vi "输入数据解析.vi"(0 "单个参数补充":dbl, 1 "从板号":dbl=1.0, 2 "主板二维码":string="BNET01", 3 "从板二维码":string="BNET01", 5 "主板引用":refnum<vi>, 7 "从板引用":refnum<vi>, 9 "主板选项":string="三级故障阀值", 11 "枚举":enum16{"主板", "从板"}(ring), 12 "快换":bool caption="快换写入") -> (4 "输出数组":dbl[][](array[numeric]), 6 "数组长度":dbl[](array[numeric]), 8 "循环次数":i32, 10 "命令":u32, 14 "名称":string[](array[string]), 15 "命令序号":u32[](array[numeric]))   [LabVIEW 2013] (continued)
              tunnel: [w18498 w18509 w18520 w18531 w18541 w18551 w18562] -> w18492
              frame 0, Default {
                # "电压过高"
                n7256 = disable-structure shown="启用" {
                  disable-tunnel: [w18504 w18507] -> w18500
                  disable-tunnel: [w18503 w18507] -> w18499
                  disable-tunnel: w18497 -> [w18502 _]
                  frame Disabled {
                    n7257 = Unbundle By Name(w18502) -> ("电压过高"=w18501:dbl)
                    n7258 = call "输入分辨率计算-EV05.vi"("1字节?"=FALSE, "数值"=w18501, "分辨率"=0.1) -> ("低字节"=w18503:dbl, "高字节1"=w18504:dbl)  [unwired: 2 in, 5 out]
                  }
                  frame Enabled {
                    w18507 = 255 ("高字节1")
                  }
                }
                n7259 = Build Array(w18500, w18499) -> (w18498:i32[])
              }
              frame 1 {
                # "电压过低"
                n7260 = disable-structure shown="启用" {
                  disable-tunnel: [w18515 w18518] -> w18511
                  disable-tunnel: [w18514 w18518] -> w18510
                  disable-tunnel: w18508 -> [w18513 _]
                  frame Disabled {
                    n7261 = Unbundle By Name(w18513) -> ("电压过低"=w18512:dbl)
                    n7262 = call "输入分辨率计算-EV05.vi"("1字节?"=FALSE, "数值"=w18512, "分辨率"=0.1) -> ("低字节"=w18514:dbl, "高字节1"=w18515:dbl)  [unwired: 2 in, 5 out]
                  }
                  frame Enabled {
                    w18518 = 255 ("高字节1")
                  }
                }
                n7263 = Build Array(w18511, w18510) -> (w18509:i32[])
              }
              frame 2 {
                # "电压不均衡"
                n7264 = disable-structure shown="启用" {
                  disable-tunnel: [w18526 w18529] -> w18522
                  disable-tunnel: [w18525 w18529] -> w18521
                  disable-tunnel: w18519 -> [w18524 _]
                  frame Disabled {
                    n7265 = Unbundle By Name(w18524) -> ("电压不均衡(V)"=w18523:dbl)
                    n7266 = call "输入分辨率计算-EV05.vi"("1字节?"=FALSE, "数值"=w18523, "分辨率"=0.1) -> ("低字节"=w18525:dbl, "高字节1"=w18526:dbl)  [unwired: 2 in, 5 out]
                  }
                  frame Enabled {
                    w18529 = 255 ("高字节1")
                  }
                }
                n7267 = Build Array(w18522, w18521) -> (w18520:i32[])
              }
              frame 3 {
                # "温度过高"
                n7268 = disable-structure shown="启用" {
                  disable-tunnel: [w18536 255 ("高字节1")] -> w18532
                  disable-tunnel: w18530 -> [w18534 _]
                  frame Disabled {
                    n7269 = Unbundle By Name(w18534) -> ("温度过高"=w18533:dbl)
                    n7270 = call "输入分辨率计算-EV05.vi"("1字节?"=TRUE, "数值"=w18533, "偏移量"=-40.0, "分辨率"=1.0) -> ("高字节1"=w18536:dbl)  [unwired: 1 in, 6 out]
                  }
                  frame Enabled {
                  }
                }
                n7271 = Build Array(w18532) -> (w18531:i32[])
              }
              frame 4 {
                # "温度过低"
                n7272 = disable-structure shown="启用" {
                  disable-tunnel: [w18546 255 ("高字节1")] -> w18542
                  disable-tunnel: w18540 -> [w18544 _]
                  frame Disabled {
                    n7273 = Unbundle By Name(w18544) -> ("温度过低"=w18543:dbl)
                    n7274 = call "输入分辨率计算-EV05.vi"("1字节?"=TRUE, "数值"=w18543, "偏移量"=-40.0, "分辨率"=1.0) -> ("高字节1"=w18546:dbl)  [unwired: 1 in, 6 out]
                  }
                  frame Enabled {
                  }
                }
                n7275 = Build Array(w18542) -> (w18541:i32[])
              }
              frame 5 {
                # "温度不均衡"
                n7276 = disable-structure shown="启用" {
                  disable-tunnel: [w18555 255 ("高字节1")] -> w18552
                  disable-tunnel: w18550 -> [w18554 _]
                  frame Disabled {
                    n7277 = Unbundle By Name(w18554) -> ("温度不均衡"=w18553:dbl)
                    n7278 = call "输入分辨率计算-EV05.vi"("1字节?"=TRUE, "数值"=w18553, "分辨率"=1.0) -> ("高字节1"=w18555:dbl)  [unwired: 2 in, 6 out]
                  }
                  frame Enabled {
                  }
                }
                n7279 = Build Array(w18552) -> (w18551:i32[])
              }
              frame 6 {
                # "SOC过低"
                n7280 = disable-structure shown="启用" {
                  disable-tunnel: w18561 -> [w18566 _]
                  disable-tunnel: [w18563 w18569] -> w18560
                  disable-tunnel: [w18564 w18569] -> w18559
                  frame Enabled {
                    n7281 = Unbundle By Name(w18566) -> ("SOC过低"=w18565:dbl)
                    n7282 = call "输入分辨率计算-EV05.vi"("1字节?"=FALSE, "数值"=w18565, "分辨率"=0.1) -> ("低字节"=w18563:dbl, "高字节1"=w18564:dbl)  [unwired: 2 in, 5 out]
                  }
                  frame Disabled {
                    w18569 = 255 ("高字节1")
                  }
                }
                n7283 = Build Array(w18559, w18560) -> (w18562:dbl[])
              }
            }
            n7284 = Insert Into Array(array=w18493, new element=w18492) -> (w18494:dbl[])  [unwired: 1 in]
          }
          n7285 = Build Array(w18487) -> (w18486:dbl[][])
        }
        frame "SOC过低(2)" {
          n7286 = Unbundle By Name(w18574) -> ("二级故障(从板)"=w18575:refnum<vi>)
          n7287 = property class="Clust (严格)"(reference=w18575) -> ("Value"=w18573:T8)  [unwired: 1 in, 2 out]
          n7288 = for {
            N: 7 -> [_]
            tunnel: w18573 -> [w18585]
            shift-right: [w18584] -> w18577
            shift-left: dbl[] [] -> [w18583]
            i -> [w18586]
            n7289 = case shown="6" w18586 {
              tunnel: w18585 -> [w18587 w18598 w18609 w18620 w18630 w18640 w18651]
              tunnel: [w18588 w18599 w18610 w18621 w18631 w18641 w18652] -> w18582
              frame 0, Default {
                # "电压过高"
                n7290 = disable-structure shown="启用" {
                  disable-tunnel: [w18594 w18597] -> w18590
                  disable-tunnel: [w18593 w18597] -> w18589
                  disable-tunnel: w18587 -> [w18592 _]
                  frame Disabled {
                    n7291 = Unbundle By Name(w18592) -> ("电压过高"=w18591:dbl)
                    n7292 = call "输入分辨率计算-EV05.vi"("1字节?"=FALSE, "数值"=w18591, "分辨率"=0.1) -> ("低字节"=w18593:dbl, "高字节1"=w18594:dbl)  [unwired: 2 in, 5 out]
                  }
                  frame Enabled {
                    w18597 = 255 ("高字节1")
                  }
                }
                n7293 = Build Array(w18590, w18589) -> (w18588:i32[])
              }
              frame 1 {
                # "电压过低"
                n7294 = disable-structure shown="启用" {
                  disable-tunnel: [w18605 w18608] -> w18601
                  disable-tunnel: [w18604 w18608] -> w18600
                  disable-tunnel: w18598 -> [w18603 _]
                  frame Disabled {
                    n7295 = Unbundle By Name(w18603) -> ("电压过低"=w18602:dbl)
                    n7296 = call "输入分辨率计算-EV05.vi"("1字节?"=FALSE, "数值"=w18602, "分辨率"=0.1) -> ("低字节"=w18604:dbl, "高字节1"=w18605:dbl)  [unwired: 2 in, 5 out]
                  }
                  frame Enabled {
                    w18608 = 255 ("高字节1")
                  }
                }
                n7297 = Build Array(w18601, w18600) -> (w18599:i32[])
              }
              frame 2 {
                # "电压不均衡"
                n7298 = disable-structure shown="启用" {
                  disable-tunnel: [w18616 w18619] -> w18612
                  disable-tunnel: [w18615 w18619] -> w18611
                  disable-tunnel: w18609 -> [w18614 _]
                  frame Disabled {
                    n7299 = Unbundle By Name(w18614) -> ("电压不均衡(V)"=w18613:dbl)
                    n7300 = call "输入分辨率计算-EV05.vi"("1字节?"=FALSE, "数值"=w18613, "分辨率"=0.1) -> ("低字节"=w18615:dbl, "高字节1"=w18616:dbl)  [unwired: 2 in, 5 out]
                  }
                  frame Enabled {
                    w18619 = 255 ("高字节1")
                  }
                }
                n7301 = Build Array(w18612, w18611) -> (w18610:i32[])
              }
              frame 3 {
                # "温度过高"
                n7302 = disable-structure shown="启用" {
                  disable-tunnel: [w18626 255 ("高字节1")] -> w18622
                  disable-tunnel: w18620 -> [w18624 _]
                  frame Disabled {
                    n7303 = Unbundle By Name(w18624) -> ("温度过高"=w18623:dbl)
                    n7304 = call "输入分辨率计算-EV05.vi"("1字节?"=TRUE, "数值"=w18623, "偏移量"=-40.0, "分辨率"=1.0) -> ("高字节1"=w18626:dbl)  [unwired: 1 in, 6 out]
                  }
                  frame Enabled {
                  }
                }
                n7305 = Build Array(w18622) -> (w18621:i32[])
              }
              frame 4 {
                # "温度过低"
                n7306 = disable-structure shown="启用" {
                  disable-tunnel: [w18636 255 ("高字节1")] -> w18632
                  disable-tunnel: w18630 -> [w18634 _]
                  frame Disabled {
                    n7307 = Unbundle By Name(w18634) -> ("温度过低"=w18633:dbl)
                    n7308 = call "输入分辨率计算-EV05.vi"("1字节?"=TRUE, "数值"=w18633, "偏移量"=-40.0, "分辨率"=1.0) -> ("高字节1"=w18636:dbl)  [unwired: 1 in, 6 out]
                  }
                  frame Enabled {
                  }
                }
                n7309 = Build Array(w18632) -> (w18631:i32[])
              }
              frame 5 {
                # "温度不均衡"
                n7310 = disable-structure shown="启用" {
                  disable-tunnel: [w18645 255 ("高字节1")] -> w18642
                  disable-tunnel: w18640 -> [w18644 _]
                  frame Disabled {
                    n7311 = Unbundle By Name(w18644) -> ("温度不均衡"=w18643:dbl)
                    n7312 = call "输入分辨率计算-EV05.vi"("1字节?"=TRUE, "数值"=w18643, "分辨率"=1.0) -> ("高字节1"=w18645:dbl)  [unwired: 2 in, 6 out]
                  }
                  frame Enabled {
                  }
                }
                n7313 = Build Array(w18642) -> (w18641:i32[])
              }
              frame 6 {
                # "SOC过低"
                n7314 = disable-structure shown="启用" {
                  disable-tunnel: w18651 -> [w18656 _]
                  disable-tunnel: [w18653 w18659] -> w18650
                  disable-tunnel: [w18654 w18659] -> w18649
                  frame Enabled {
                    n7315 = Unbundle By Name(w18656) -> ("SOC过低"=w18655:dbl)
                    n7316 = call "输入分辨率计算-EV05.vi"("1字节?"=FALSE, "数值"=w18655, "分辨率"=0.1) -> ("低字节"=w18653:dbl, "高字节1"=w18654:dbl)  [unwired: 2 in, 5 out]
                  }
                  frame Disabled {
                    w18659 = 255 ("高字节1")
                  }
                }
                n7317 = Build Array(w18649, w18650) -> (w18652:dbl[])
              }
            }
            n7318 = Insert Into Array(array=w18583, new element=w18582) -> (w18584:dbl[])  [unwired: 1 in]
          }
          n7319 = Build Array(w18577) -> (w18576:dbl[][])
        }
        frame "SOC过低(3)" {
          n7320 = Unbundle By Name(w18664) -> ("三级故障(从板)"=w18665:refnum<vi>)
          n7321 = property class="Clust (严格)"(reference=w18665) -> ("Value"=w18663:T8)  [unwired: 1 in, 2 out]
          n7322 = for {
            N: 7 -> [_]
            tunnel: w18663 -> [w18675]
            shift-right: [w18674] -> w18667
            shift-left: dbl[] [] -> [w18673]
            i -> [w18676]
            n7323 = case shown="6" w18676 {
              tunnel: w18675 -> [w18677 w18688 w18699 w18710 w18720 w18730 w18741]
              tunnel: [w18678 w18689 w18700 w18711 w18721 w18731 w18742] -> w18672
              frame 0, Default {
                # "电压过高"
                n7324 = disable-structure shown="启用" {
                  disable-tunnel: [w18684 w18687] -> w18680
                  disable-tunnel: [w18683 w18687] -> w18679
                  disable-tunnel: w18677 -> [w18682 _]
                  frame Disabled {
                    n7325 = Unbundle By Name(w18682) -> ("电压过高"=w18681:dbl)
                    n7326 = call "输入分辨率计算-EV05.vi"("1字节?"=FALSE, "数值"=w18681, "分辨率"=0.1) -> ("低字节"=w18683:dbl, "高字节1"=w18684:dbl)  [unwired: 2 in, 5 out]
                  }
                  frame Enabled {
                    w18687 = 255 ("高字节1")
                  }
                }
                n7327 = Build Array(w18680, w18679) -> (w18678:i32[])
              }
              frame 1 {
                # "电压过低"
                n7328 = disable-structure shown="启用" {
                  disable-tunnel: [w18695 w18698] -> w18691
                  disable-tunnel: [w18694 w18698] -> w18690
                  disable-tunnel: w18688 -> [w18693 _]
                  frame Disabled {
                    n7329 = Unbundle By Name(w18693) -> ("电压过低"=w18692:dbl)
                    n7330 = call "输入分辨率计算-EV05.vi"("1字节?"=FALSE, "数值"=w18692, "分辨率"=0.1) -> ("低字节"=w18694:dbl, "高字节1"=w18695:dbl)  [unwired: 2 in, 5 out]
                  }
                  frame Enabled {
                    w18698 = 255 ("高字节1")
                  }
                }
                n7331 = Build Array(w18691, w18690) -> (w18689:i32[])
              }
              frame 2 {
                # "电压不均衡"
                n7332 = disable-structure shown="启用" {
                  disable-tunnel: [w18706 w18709] -> w18702
                  disable-tunnel: [w18705 w18709] -> w18701
                  disable-tunnel: w18699 -> [w18704 _]
                  frame Disabled {
                    n7333 = Unbundle By Name(w18704) -> ("电压不均衡(V)"=w18703:dbl)
                    n7334 = call "输入分辨率计算-EV05.vi"("1字节?"=FALSE, "数值"=w18703, "分辨率"=0.1) -> ("低字节"=w18705:dbl, "高字节1"=w18706:dbl)  [unwired: 2 in, 5 out]
                  }
                  frame Enabled {
                    w18709 = 255 ("高字节1")
                  }
                }
                n7335 = Build Array(w18702, w18701) -> (w18700:i32[])
              }
              frame 3 {
                # "温度过高"
                n7336 = disable-structure shown="启用" {
                  disable-tunnel: [w18716 255 ("高字节1")] -> w18712
                  disable-tunnel: w18710 -> [w18714 _]
                  frame Disabled {
                    n7337 = Unbundle By Name(w18714) -> ("温度过高"=w18713:dbl)
                    n7338 = call "输入分辨率计算-EV05.vi"("1字节?"=TRUE, "数值"=w18713, "偏移量"=-40.0, "分辨率"=1.0) -> ("高字节1"=w18716:dbl)  [unwired: 1 in, 6 out]
                  }
                  frame Enabled {
                  }
                }
                n7339 = Build Array(w18712) -> (w18711:i32[])
              }
              frame 4 {
                # "温度过低"
                n7340 = disable-structure shown="启用" {
                  disable-tunnel: [w18726 255 ("高字节1")] -> w18722
                  disable-tunnel: w18720 -> [w18724 _]
                  frame Disabled {
                    n7341 = Unbundle By Name(w18724) -> ("温度过低"=w18723:dbl)
                    n7342 = call "输入分辨率计算-EV05.vi"("1字节?"=TRUE, "数值"=w18723, "偏移量"=-40.0, "分辨率"=1.0) -> ("高字节1"=w18726:dbl)  [unwired: 1 in, 6 out]
                  }
                  frame Enabled {
                  }
                }
                n7343 = Build Array(w18722) -> (w18721:i32[])
              }
              frame 5 {
                # "温度不均衡"
                n7344 = disable-structure shown="启用" {
                  disable-tunnel: [w18735 255 ("高字节1")] -> w18732
                  disable-tunnel: w18730 -> [w18734 _]
                  frame Disabled {
                    n7345 = Unbundle By Name(w18734) -> ("温度不均衡"=w18733:dbl)
                    n7346 = call "输入分辨率计算-EV05.vi"("1字节?"=TRUE, "数值"=w18733, "分辨率"=1.0) -> ("高字节1"=w18735:dbl)  [unwired: 2 in, 6 out]
                  }
                  frame Enabled {
                  }
                }
                n7347 = Build Array(w18732) -> (w18731:i32[])
              }
              frame 6 {
                # "SOC过低"
                n7348 = disable-structure shown="启用" {
                  disable-tunnel: w18741 -> [w18746 _]
                  disable-tunnel: [w18743 w18749] -> w18740
                  disable-tunnel: [w18744 w18749] -> w18739
                  frame Enabled {
                    n7349 = Unbundle By Name(w18746) -> ("SOC过低"=w18745:dbl)
                    n7350 = call "输入分辨率计算-EV05.vi"("1字节?"=FALSE, "数值"=w18745, "分辨率"=0.1) -> ("低字节"=w18743:dbl, "高字节1"=w18744:dbl)  [unwired: 2 in, 5 out]
                  }
                  frame Disabled {
                    w18749 = 255 ("高字节1")
                  }
                }
                n7351 = Build Array(w18739, w18740) -> (w18742:dbl[])
              }
            }
            n7352 = Insert Into Array(array=w18673, new element=w18672) -> (w18674:dbl[])  [unwired: 1 in]
          }
          n7353 = Build Array(w18667) -> (w18666:dbl[][])
        }
        frame "二级故障阀值" {
          n7354 = Unbundle By Name(w18754) -> ("二级故障(从板)"=w18755:refnum<vi>)
          n7355 = property class="Clust (严格)"(reference=w18755) -> ("Value"=w18753:T8)  [unwired: 1 in, 2 out]
          n7356 = for {
            N: 7 -> [_]
            tunnel: w18753 -> [w18765]
            shift-right: [w18764] -> w18757
            shift-left: dbl[] [] -> [w18763]
            i -> [w18766]
            n7357 = case shown="5" w18766 {
              tunnel: w18765 -> [w18768 w18775 w18782 w18789 w18796 w18803 w18811]
              tunnel: [w18769 w18776 w18783 w18791 w18798 w18804 w18812] -> w18762
              frame 0, Default {
                # "电压过高"
                n7358 = Unbundle By Name(w18768) -> ("电压过高"=w18767:dbl)
                n7359 = call "输入分辨率计算-EV05.vi"("1字节?"=FALSE, "数值"=w18767, "分辨率"=0.001) -> ("低字节"=w18770:dbl, "高字节1"=w18771:dbl)  [unwired: 2 in, 5 out]
                n7360 = Build Array(w18771, w18770) -> (w18769:dbl[])
              }
              frame 1 {
                # "电压过低"
                n7361 = Unbundle By Name(w18775) -> ("电压过低"=w18774:dbl)
                n7362 = call "输入分辨率计算-EV05.vi"("1字节?"=FALSE, "数值"=w18774, "分辨率"=0.001) -> ("低字节"=w18777:dbl, "高字节1"=w18778:dbl)  [unwired: 2 in, 5 out]
                n7363 = Build Array(w18778, w18777) -> (w18776:dbl[])
              }
              frame 2 {
                # "电压不均衡"
                n7364 = Unbundle By Name(w18782) -> ("电压不均衡(V)"=w18781:dbl)
                n7365 = call "输入分辨率计算-EV05.vi"("1字节?"=FALSE, "数值"=w18781, "分辨率"=0.001) -> ("低字节"=w18784:dbl, "高字节1"=w18785:dbl)  [unwired: 2 in, 5 out]
                n7366 = Build Array(w18785, w18784) -> (w18783:dbl[])
              }
              frame 3 {
                # "温度不均衡"
                n7367 = Unbundle By Name(w18789) -> ("温度过高"=w18788:dbl)
                n7368 = call "输入分辨率计算-EV05.vi"("1字节?"=TRUE, "数值"=w18788, "偏移量"=-40.0, "分辨率"=1.0) -> ("高字节1"=w18792:dbl)  [unwired: 1 in, 6 out]
                n7369 = Build Array(w18792) -> (w18791:dbl[])
              }
              frame 4 {
                # "温度过低"
                n7370 = Unbundle By Name(w18796) -> ("温度过低"=w18795:dbl)
                n7371 = call "输入分辨率计算-EV05.vi"("1字节?"=TRUE, "数值"=w18795, "偏移量"=-40.0, "分辨率"=1.0) -> ("高字节1"=w18799:dbl)  [unwired: 1 in, 6 out]
                n7372 = Build Array(w18799) -> (w18798:dbl[])
              }
              frame 5 {
                # "温度不均衡"
                n7373 = Unbundle By Name(w18803) -> ("温度不均衡"=w18802:dbl)
                n7374 = call "输入分辨率计算-EV05.vi"("1字节?"=TRUE, "数值"=w18802, "分辨率"=1.0) -> ("高字节1"=w18805:dbl)  [unwired: 2 in, 6 out]
                n7375 = Build Array(w18805) -> (w18804:dbl[])
              }
              frame 6 {
                # "SOC过低"
                n7376 = Unbundle By Name(w18811) -> ("SOC过低"=w18810:dbl)
                n7377 = call "输入分辨率计算-EV05.vi"("1字节?"=FALSE, "数值"=w18810, "分辨率"=0.1) -> ("低字节"=w18808:dbl, "高字节1"=w18809:dbl)  [unwired: 2 in, 5 out]
                n7378 = Build Array(w18809, w18808) -> (w18812:dbl[])
              }
            }
            n7379 = Insert Into Array(array=w18763, new element=w18762) -> (w18764:dbl[])  [unwired: 1 in]
          }
          n7380 = Build Array(w18757) -> (w18756:dbl[][])
        }
        frame "三级故障阀值" {
          n7381 = Unbundle By Name(w18819) -> ("三级故障(从板)"=w18820:refnum<vi>)
          n7382 = property class="Clust (严格)"(reference=w18820) -> ("Value"=w18818:T8)  [unwired: 1 in, 2 out]
          n7383 = for {
            N: 7 -> [_]
            tunnel: w18818 -> [w18830]
            shift-right: [w18829] -> w18822
            shift-left: dbl[] [] -> [w18828]
            i -> [w18831]
            n7384 = case shown="2" w18831 {
              tunnel: w18830 -> [w18833 w18840 w18847 w18854 w18861 w18868 w18876]
              tunnel: [w18834 w18841 w18848 w18856 w18863 w18869 w18877] -> w18827
              frame 0, Default {
                # "电压过高"
                n7385 = Unbundle By Name(w18833) -> ("电压过高"=w18832:dbl)
                n7386 = call "输入分辨率计算-EV05.vi"("1字节?"=FALSE, "数值"=w18832, "分辨率"=0.001) -> ("低字节"=w18835:dbl, "高字节1"=w18836:dbl)  [unwired: 2 in, 5 out]
                n7387 = Build Array(w18836, w18835) -> (w18834:dbl[])
              }
              frame 1 {
                # "电压过低"
                n7388 = Unbundle By Name(w18840) -> ("电压过低"=w18839:dbl)
                n7389 = call "输入分辨率计算-EV05.vi"("1字节?"=FALSE, "数值"=w18839, "分辨率"=0.001) -> ("低字节"=w18842:dbl, "高字节1"=w18843:dbl)  [unwired: 2 in, 5 out]
                n7390 = Build Array(w18843, w18842) -> (w18841:dbl[])
              }
              frame 2 {
                # "电压不均衡"
                n7391 = Unbundle By Name(w18847) -> ("电压不均衡(V)"=w18846:dbl)
                n7392 = call "输入分辨率计算-EV05.vi"("1字节?"=FALSE, "数值"=w18846, "分辨率"=0.001) -> ("低字节"=w18849:dbl, "高字节1"=w18850:dbl)  [unwired: 2 in, 5 out]
                n7393 = Build Array(w18850, w18849) -> (w18848:dbl[])
              }
              frame 3 {
                # "温度不均衡"
                n7394 = Unbundle By Name(w18854) -> ("温度过高"=w18853:dbl)
                n7395 = call "输入分辨率计算-EV05.vi"("1字节?"=TRUE, "数值"=w18853, "偏移量"=-40.0, "分辨率"=1.0) -> ("高字节1"=w18857:dbl)  [unwired: 1 in, 6 out]
                n7396 = Build Array(w18857) -> (w18856:dbl[])
              }
              frame 4 {
                # "温度过低"
                n7397 = Unbundle By Name(w18861) -> ("温度过低"=w18860:dbl)
                n7398 = call "输入分辨率计算-EV05.vi"("1字节?"=TRUE, "数值"=w18860, "偏移量"=-40.0, "分辨率"=1.0) -> ("高字节1"=w18864:dbl)  [unwired: 1 in, 6 out]
                n7399 = Build Array(w18864) -> (w18863:dbl[])
              }
              frame 5 {
                # "温度不均衡"
                n7400 = Unbundle By Name(w18868) -> ("温度不均衡"=w18867:dbl)
                n7401 = call "输入分辨率计算-EV05.vi"("1字节?"=TRUE, "数值"=w18867, "分辨率"=1.0) -> ("高字节1"=w18870:dbl)  [unwired: 2 in, 6 out]
                n7402 = Build Array(w18870) -> (w18869:dbl[])
              }
              frame 6 {
                # "SOC过低"
                n7403 = Unbundle By Name(w18876) -> ("SOC过低"=w18875:dbl)
                n7404 = call "输入分辨率计算-EV05.vi"("1字节?"=FALSE, "数值"=w18875, "分辨率"=0.1) -> ("低字节"=w18873:dbl, "高字节1"=w18874:dbl)  [unwired: 2 in, 5 out]
                n7405 = Build Array(w18874, w18873) -> (w18877:dbl[])
              }
            }
            n7406 = Insert Into Array(array=w18828, new element=w18827) -> (w18829:dbl[])  [unwired: 1 in]
          }
          n7407 = Build Array(w18822) -> (w18821:dbl[][])
        }
        frame "快换参数" {
          n7408 = case shown="真" w18883 {
            tunnel: [_ w18896] -> w18887
            tunnel: [_ w18895] -> w18886
            tunnel: w18885 -> [_ w18891]
            tunnel: [_ w18894] -> w18884
            tunnel: [_ u32 35 ("命令序号")] -> w18882
            tunnel: [_ w18889] -> w18881
            tunnel: [_ w18888] -> w18880
            frame False {
            }
            frame True {
              w18889 = 7
              n7409 = Unbundle By Name(w18891) -> ("电池组信息(从板)"=w18892:refnum<vi>)
              n7410 = property class="Clust (严格)"(reference=w18892) -> ("Value"=w18890:T9)  [unwired: 1 in, 2 out]
              n7411 = for {
                N: w18889 -> [_]
                tunnel: [w18902] -> w18896 mode=indexing
                tunnel: [w18901] -> w18895 mode=indexing
                tunnel: w18890 -> [w18900]
                tunnel: [w18899] -> w18894 mode=indexing
                tunnel: [w18897] -> w18888 mode=indexing
                i -> [w18898]
                n7412 = case shown="3" w18898 {
                  tunnel: [30 ("单个参数补充") 4 ("单个参数补充") 8 ("单个参数补充") 6 ("单个参数补充") 4 ("单个参数补充") 8 ("单个参数补充") 14 ("单个参数补充")] -> w18902
                  tunnel: [u32 1 ("命令序号") u32 2 ("命令序号") u32 3 ("命令序号") u32 4 ("命令序号") u32 5 ("命令序号") u32 6 ("命令序号") u32 7 ("命令序号")] -> w18901
                  tunnel: w18900 -> [w18906 w18981 w18989 w19019 w19030 w19038 w19059]
                  tunnel: [w18903 w18974 w19006 w19021 w19031 w19036 w19061] -> w18899
                  tunnel: ["电池包信息1" "电池包序号" "充放电安时" "充电次数时间" "SOC" "车牌号" "充电参数"] -> w18897
                  frame 0, Default {
                    w18916 = ":" ("正则表达式")
                    w18924 = 0.0 ("元素")
                    w18943 = 256.0 ("y")
                    w18948 = 256.0 ("y")
                    w18961 = 2 ("偏移量(0)")
                    w18958 = "-" ("正则表达式")
                    # "电池组信息"
                    n7413 = Unbundle By Name(w18906) -> ("串联数"=w18965:dbl, "并联数"=w18964:dbl, "电池厂家"=w18904:dbl, "电池类型"=w18905:dbl, "生产日期"=w18963:string)
                    n7414 = Unbundle By Name(w18906) -> ("额定能量"=w18929:dbl, "额定容量"=w18931:dbl, "实际容量"=w18930:dbl, "额定总压"=w18954:dbl)
                    n7415 = Match Pattern(string=w18963, regular expression=w18958) -> (before substring=w18962:string, after substring=w18959:string)  [unwired: 3 out]
                    n7416 = Match Pattern(string=w18959, regular expression=w18958) -> (before substring=w18957:string, after substring=w18922:string)  [unwired: 3 out]
                    n7417 = Match Pattern(string=w18922, regular expression=" " ("正则表达式")) -> (before substring=w18920:string, after substring=w18919:string)  [unwired: 3 out]
                    n7418 = call "输入分辨率计算-EV05.vi"("1字节?"=FALSE, "数值"=w18929, "分辨率"=0.1) -> ("低字节"=w18928:dbl, "高字节1"=w18927:dbl)  [unwired: 2 in, 5 out]
                    n7419 = String Subset(string=w18962, offset (0)=w18961, length (rest)=w18961) -> (substring=w18960:string)
                    n7420 = call "输入分辨率计算-EV05.vi"("1字节?"=TRUE, "数值 2"=w18930, "数值"=w18931, "分辨率"=0.001) -> ("高字节 2"=w18932:dbl, "高字节1"=w18933:dbl)  [unwired: 1 in, 5 out]
                    n7421 = Match Pattern(string=w18919, regular expression=w18916) -> (before substring=w18918:string, after substring=w18917:string)  [unwired: 3 out]
                    n7422 = Fract/Exp String To Number(string=w18960) -> (number=w18912:dbl)  [unwired: 1 in, 3 out]
                    n7423 = Fract/Exp String To Number(string=w18957) -> (number=w18911:dbl)  [unwired: 4 out]
                    n7424 = Fract/Exp String To Number(string=w18920) -> (number=w18910:dbl)  [unwired: 4 out]
                    n7425 = Match Pattern(string=w18917, regular expression=w18916) -> (before substring=w18915:string, after substring=w18914:string)  [unwired: 3 out]
                    n7426 = call "输入分辨率计算-EV05.vi"("1字节?"=FALSE, "数值"=w18954, "分辨率"=0.1) -> ("低字节"=w18925:dbl, "高字节1"=w18926:dbl)  [unwired: 2 in, 5 out]
                    n7427 = Quotient & Remainder(x=w18933, y=w18948) -> (x-y*floor(x/y)=w18947:dbl, floor(x/y)=w18951:dbl)
                    n7428 = Fract/Exp String To Number(string=w18918) -> (number=w18909:dbl)  [unwired: 4 out]
                    n7429 = Quotient & Remainder(x=w18932, y=w18943) -> (x-y*floor(x/y)=w18939:dbl, floor(x/y)=w18940:dbl)
                    n7430 = Quotient & Remainder(x=w18951, y=w18948) -> (x-y*floor(x/y)=w18946:dbl, floor(x/y)=w18950:dbl)
                    n7431 = Fract/Exp String To Number(string=w18915) -> (number=w18908:dbl)  [unwired: 4 out]
                    n7432 = Quotient & Remainder(x=w18940, y=w18943) -> (x-y*floor(x/y)=w18938:dbl, floor(x/y)=w18941:dbl)
                    n7433 = call <vilib>:"Trim Whitespace.vi"("string"=w18914) -> ("trimmed string"=w18913:string)  [unwired: 1 in]
                    n7434 = Quotient & Remainder(x=w18950, y=w18948) -> (x-y*floor(x/y)=w18945:dbl, floor(x/y)=w18949:dbl)
                    n7435 = Quotient & Remainder(x=w18941, y=w18943) -> (x-y*floor(x/y)=w18937:dbl, floor(x/y)=w18942:dbl)
                    n7436 = Quotient & Remainder(x=w18965, y=256.0) -> (x-y*floor(x/y)=w18967:dbl, floor(x/y)=w18968:dbl)
                    n7437 = Fract/Exp String To Number(string=w18913) -> (number=w18907:dbl)  [unwired: 4 out]
                    n7438 = Quotient & Remainder(x=w18949, y=w18948) -> (x-y*floor(x/y)=w18944:dbl)  [unwired: 1 out]
                    n7439 = Quotient & Remainder(x=w18942, y=w18943) -> (x-y*floor(x/y)=w18936:dbl)  [unwired: 1 out]
                    n7440 = Build Array(w18927, w18928, w18944, w18945, w18946, w18947, w18936, w18937, w18938, w18939, w18926, w18925, w18924, w18924, w18924, w18912, w18911, w18910, w18909, w18908, w18907) -> (w18923:dbl[])
                    n7441 = Build Array(w18968, w18967, w18964, w18904, w18905) -> (w18966:dbl[])
                    n7442 = Insert Into Array(array=w18966, new element=w18923) -> (w18903:dbl[])  [unwired: 1 in]
                  }
                  frame 1 {
                    n7443 = Unbundle By Name(w18981) -> ("电池包序号"=w18978:dbl)
                    n7444 = Quotient & Remainder(x=w18978, y=256.0) -> (x-y*floor(x/y)=w18975:dbl, floor(x/y)=w18976:dbl)
                    n7445 = Build Array(w18976, w18975) -> (w18974:dbl[])
                  }
                  frame 2 {
                    w18997 = 256.0 ("y")
                    w19002 = 256.0 ("y")
                    # "充放电安时/安时数"
                    n7446 = Unbundle By Name(w18989) -> ("充电总安时"=w18986:dbl, "放电总这时"=w18985:dbl)
                    n7447 = call "输入分辨率计算-EV05.vi"("1字节?"=TRUE, "数值 2"=w18985, "数值"=w18986, "分辨率"=0.001) -> ("高字节 2"=w18983:dbl, "高字节1"=w18984:dbl)  [unwired: 1 in, 5 out]
                    n7448 = Quotient & Remainder(x=w18984, y=w19002) -> (x-y*floor(x/y)=w19001:dbl, floor(x/y)=w19005:dbl)
                    n7449 = Quotient & Remainder(x=w18983, y=w18997) -> (x-y*floor(x/y)=w18993:dbl, floor(x/y)=w18994:dbl)
                    n7450 = Quotient & Remainder(x=w19005, y=w19002) -> (x-y*floor(x/y)=w19000:dbl, floor(x/y)=w19004:dbl)
                    n7451 = Quotient & Remainder(x=w18994, y=w18997) -> (x-y*floor(x/y)=w18992:dbl, floor(x/y)=w18995:dbl)
                    n7452 = Quotient & Remainder(x=w19004, y=w19002) -> (x-y*floor(x/y)=w18999:dbl, floor(x/y)=w19003:dbl)
                    n7453 = Quotient & Remainder(x=w18995, y=w18997) -> (x-y*floor(x/y)=w18991:dbl, floor(x/y)=w18996:dbl)
                    n7454 = Quotient & Remainder(x=w19003, y=w19002) -> (x-y*floor(x/y)=w18998:dbl)  [unwired: 1 out]
                    n7455 = Quotient & Remainder(x=w18996, y=w18997) -> (x-y*floor(x/y)=w18990:dbl)  [unwired: 1 out]
                    n7456 = Build Array(w18998, w18999, w19000, w19001, w18990, w18991, w18992, w18993) -> (w19006:dbl[])
                  }
                  frame 3 {
                    w19014 = 256.0 ("y")
                    # "充电次数"
                    n7457 = Unbundle By Name(w19019) -> ("放空次数"=w19018:dbl, "充满次数"=w19016:dbl, "充电次数"=w19015:dbl)
                    n7458 = Quotient & Remainder(x=w19018, y=w19014) -> (x-y*floor(x/y)=w19020:dbl, floor(x/y)=w19017:dbl)
                    n7459 = Quotient & Remainder(x=w19016, y=w19014) -> (x-y*floor(x/y)=w19012:dbl, floor(x/y)=w19013:dbl)
                    n7460 = Quotient & Remainder(x=w19015, y=w19014) -> (x-y*floor(x/y)=w19010:dbl, floor(x/y)=w19011:dbl)
                    n7461 = Build Array(w19017, w19020, w19013, w19012, w19011, w19010) -> (w19021:dbl[])
                  }
                  frame 4 {
                    # "SOC"
                    n7462 = Unbundle By Name(w19030) -> ("SOC"=w19029:dbl)
                    n7463 = call "输入分辨率计算-EV05.vi"("1字节?"=FALSE, "数值"=w19029, "分辨率"=0.1) -> ("低字节"=w19025:dbl, "高字节1"=w19026:dbl)  [unwired: 2 in, 5 out]
                    n7464 = Build Array(w19026, w19025) -> (w19031:dbl[])
                  }
                  frame 5 {
                    # "车牌号"
                    n7465 = Unbundle By Name(w19038) -> ("车牌号"=w19037:string)
                    n7466 = String To Byte Array(string=w19037) -> (unsigned byte array=w19041:u8[])
                    n7467 = Array Subset(array=w19041, length=8 ("长度")) -> (w19036:u8[])  [unwired: 1 in]
                  }
                  frame 6 {
                    n7468 = Unbundle By Name(w19059) -> ("最大允许单体电压"=w19057:dbl, "最大允许总电压"=w19056:dbl, "最大允许温度"=w19055:dbl, "最小允许温度"=w19054:dbl, "最大允许充电电流"=w19053:dbl, "最小允许充电电流"=w19052:dbl, "电流步长"=w19048:dbl, "最小允许单体电压"=w19051:dbl)
                    n7469 = call "输入分辨率计算-EV05.vi"("1字节?"=FALSE, "数值 2"=w19051, "数值"=w19057, "分辨率"=0.001) -> ("低字节 2"=w19043:dbl, "高字节 2"=w19044:dbl, "低字节"=w19067:dbl, "高字节1"=w19068:dbl)  [unwired: 1 in, 3 out]
                    n7470 = call "输入分辨率计算-EV05.vi"("1字节?"=FALSE, "数值"=w19056, "分辨率"=0.1) -> ("低字节"=w19065:dbl, "高字节1"=w19066:dbl)  [unwired: 2 in, 5 out]
                    n7471 = call "输入分辨率计算-EV05.vi"("1字节?"=TRUE, "数值 2"=w19054, "数值"=w19055, "偏移量"=-40.0, "分辨率"=1.0) -> ("高字节 2"=w19060:dbl, "高字节1"=w19064:dbl)  [unwired: 5 out]
                    n7472 = call "输入分辨率计算-EV05.vi"("1字节?"=FALSE, "数值 2"=w19052, "数值"=w19053, "偏移量"=0.0, "分辨率"=0.1) -> ("低字节 2"=w19049:dbl, "高字节 2"=w19050:dbl, "低字节"=w19062:dbl, "高字节1"=w19063:dbl)  [unwired: 3 out]
                    n7473 = Quotient & Remainder(x=w19048, y=256.0) -> (x-y*floor(x/y)=w19045:dbl, floor(x/y)=w19046:dbl)
                    n7474 = Build Array(w19068, w19067, w19066, w19065, w19064, w19060, w19063, w19062, w19050, w19049, w19046, w19045, w19044, w19043) -> (w19061:dbl[])
                  }
                }
              }
            }
          }
        }
        frame "均衡参数" {
          w19083 = 2
          n7475 = Unbundle By Name(w19086) -> ("均衡参数"=w19081:refnum<vi>)
          n7476 = property class="Clust (严格)"(reference=w19081) -> ("Value"=w19080:T10)  [unwired: 1 in, 2 out]
          n7477 = for {
            N: w19083 -> [_]
            tunnel: [w19094] -> w19088 mode=indexing
            tunnel: [w19093] -> w19087 mode=indexing
            tunnel: w19080 -> [w19092]
            tunnel: [w19091] -> w19085 mode=indexing
            tunnel: [w19089] -> w19082 mode=indexing
            i -> [w19090]
            n7478 = case shown="0, 默认" w19090 {
              tunnel: [24 ("命令序号") 22 ("单个参数补充")] -> w19094
              tunnel: [u32 1 ("命令序号") u32 2 ("命令序号")] -> w19093
              tunnel: w19092 -> [w19125 w19178]
              tunnel: [w19124 w19150] -> w19091
              tunnel: ["均衡阀值" "充电结束电压"] -> w19089
              frame 0, Default {
                n7479 = Unbundle By Name(w19125) -> ("均衡计算-电压高阀值2级"=w19115:sgl, "均衡计算-电压高阀值1级"=w19114:sgl, "均衡计算-电压低阀值1级"=w19113:sgl, "均衡计算-电压低阀值2级"=w19112:sgl, "均衡计算-最低电压阀值"=w19111:sgl, "均衡停止-最低电压阀值"=w19110:sgl, "均衡计算-电压极差阀值"=w19109:sgl)
                n7480 = call "输入分辨率计算-EV05.vi"("1字节?"=FALSE, "数值"=w19109, "分辨率"=0.001) -> ("低字节"=w19095:dbl, "高字节1"=w19096:dbl)  [unwired: 2 in, 5 out]
                n7481 = call "输入分辨率计算-EV05.vi"("1字节?"=FALSE, "数值 2"=w19110, "数值"=w19111, "分辨率"=0.001) -> ("低字节 2"=w19097:dbl, "高字节 2"=w19098:dbl, "低字节"=w19099:dbl, "高字节1"=w19100:dbl)  [unwired: 1 in, 3 out]
                n7482 = call "输入分辨率计算-EV05.vi"("1字节?"=FALSE, "数值 2"=w19114, "数值"=w19115, "分辨率"=0.001) -> ("低字节 2"=w19105:dbl, "高字节 2"=w19106:dbl, "低字节"=w19107:dbl, "高字节1"=w19108:dbl)  [unwired: 1 in, 3 out]
                n7483 = call "输入分辨率计算-EV05.vi"("1字节?"=FALSE, "数值 2"=w19112, "数值"=w19113, "分辨率"=0.001) -> ("低字节 2"=w19101:dbl, "高字节 2"=w19102:dbl, "低字节"=w19103:dbl, "高字节1"=w19104:dbl)  [unwired: 1 in, 3 out]
                n7484 = Build Array(w19108, w19107, w19106, w19105, w19104, w19103, w19102, w19101, w19100, w19099, w19098, w19097, w19096, w19095) -> (w19124:dbl[])
              }
              frame 1 {
                n7485 = Unbundle By Name(w19178) -> ("充电结束电压(90%)"=w19162:sgl, "充电结束电压(91%)"=w19161:sgl, "充电结束电压(92%)"=w19160:sgl, "充电结束电压(93%)"=w19159:sgl, "充电结束电压(94%)"=w19158:sgl, "充电结束电压(95%)"=w19157:sgl, "充电结束电压(96%)"=w19156:sgl, "充电结束电压(97%)"=w19155:sgl, "充电结束电压(98%)"=w19154:sgl, "充电结束电压(99%)"=w19153:sgl, "充电结束电压(100%)"=w19152:sgl)
                n7486 = call "输入分辨率计算-EV05.vi"("1字节?"=FALSE, "数值 2"=w19159, "数值"=w19160, "分辨率"=0.001) -> ("低字节 2"=w19143:dbl, "高字节 2"=w19144:dbl, "低字节"=w19145:dbl, "高字节1"=w19146:dbl)  [unwired: 1 in, 3 out]
                n7487 = call "输入分辨率计算-EV05.vi"("1字节?"=FALSE, "数值 2"=w19157, "数值"=w19158, "分辨率"=0.001) -> ("低字节 2"=w19139:dbl, "高字节 2"=w19140:dbl, "低字节"=w19141:dbl, "高字节1"=w19142:dbl)  [unwired: 1 in, 3 out]
                n7488 = call "输入分辨率计算-EV05.vi"("1字节?"=FALSE, "数值"=w19152, "分辨率"=0.001) -> ("低字节"=w19129:dbl, "高字节1"=w19130:dbl)  [unwired: 2 in, 5 out]
                n7489 = call "输入分辨率计算-EV05.vi"("1字节?"=FALSE, "数值 2"=w19153, "数值"=w19154, "分辨率"=0.001) -> ("低字节 2"=w19131:dbl, "高字节 2"=w19132:dbl, "低字节"=w19133:dbl, "高字节1"=w19134:dbl)  [unwired: 1 in, 3 out]
                n7490 = call "输入分辨率计算-EV05.vi"("1字节?"=FALSE, "数值 2"=w19161, "数值"=w19162, "分辨率"=0.001) -> ("低字节 2"=w19147:dbl, "高字节 2"=w19148:dbl, "低字节"=w19149:dbl, "高字节1"=w19151:dbl)  [unwired: 1 in, 3 out]
                n7491 = call "输入分辨率计算-EV05.vi"("1字节?"=FALSE, "数值 2"=w19155, "数值"=w19156, "分辨率"=0.001) -> ("低字节 2"=w19135:dbl, "高字节 2"=w19136:dbl, "低字节"=w19137:dbl, "高字节1"=w19138:dbl)  [unwired: 1 in, 3 out]
                n7492 = Build Array(w19151, w19149, w19148, w19147, w19146, w19145, w19144, w19143, w19142, w19141, w19140, w19139, w19138, w19137, w19136, w19135, w19134, w19133, w19132, w19131, w19130, w19129) -> (w19150:dbl[])
              }
            }
          }
        }
        frame "均衡阀值" {
          w19182 = 1
          n7493 = Unbundle By Name(w19185) -> ("均衡参数"=w19180:refnum<vi>)
          n7494 = property class="Clust (严格)"(reference=w19180) -> ("Value"=w19179:T10)  [unwired: 1 in, 2 out]
          n7495 = for {
            N: w19182 -> [_]
            tunnel: [w19193] -> w19187 mode=indexing
            tunnel: [w19192] -> w19186 mode=indexing
            tunnel: w19179 -> [w19191]
            tunnel: [w19190] -> w19184 mode=indexing
            tunnel: [w19188] -> w19181 mode=indexing
            i -> [w19189]
            n7496 = case shown="0, 默认" w19189 {
              tunnel: [24 ("命令序号") 22 ("单个参数补充")] -> w19193
              tunnel: [u32 1 ("命令序号") u32 2 ("命令序号")] -> w19192
              tunnel: w19191 -> [w19224 w19277]
              tunnel: [w19223 w19249] -> w19190
              tunnel: ["均衡阀值" "充电结束电压"] -> w19188
              frame 0, Default {
                n7497 = Unbundle By Name(w19224) -> ("均衡计算-电压高阀值2级"=w19214:sgl, "均衡计算-电压高阀值1级"=w19213:sgl, "均衡计算-电压低阀值1级"=w19212:sgl, "均衡计算-电压低阀值2级"=w19211:sgl, "均衡计算-最低电压阀值"=w19210:sgl, "均衡停止-最低电压阀值"=w19209:sgl, "均衡计算-电压极差阀值"=w19208:sgl)
                n7498 = call "输入分辨率计算-EV05.vi"("1字节?"=FALSE, "数值"=w19208, "分辨率"=0.001) -> ("低字节"=w19194:dbl, "高字节1"=w19195:dbl)  [unwired: 2 in, 5 out]
                n7499 = call "输入分辨率计算-EV05.vi"("1字节?"=FALSE, "数值 2"=w19209, "数值"=w19210, "分辨率"=0.001) -> ("低字节 2"=w19196:dbl, "高字节 2"=w19197:dbl, "低字节"=w19198:dbl, "高字节1"=w19199:dbl)  [unwired: 1 in, 3 out]
                n7500 = call "输入分辨率计算-EV05.vi"("1字节?"=FALSE, "数值 2"=w19213, "数值"=w19214, "分辨率"=0.001) -> ("低字节 2"=w19204:dbl, "高字节 2"=w19205:dbl, "低字节"=w19206:dbl, "高字节1"=w19207:dbl)  [unwired: 1 in, 3 out]
                n7501 = call "输入分辨率计算-EV05.vi"("1字节?"=FALSE, "数值 2"=w19211, "数值"=w19212, "分辨率"=0.001) -> ("低字节 2"=w19200:dbl, "高字节 2"=w19201:dbl, "低字节"=w19202:dbl, "高字节1"=w19203:dbl)  [unwired: 1 in, 3 out]
                n7502 = Build Array(w19207, w19206, w19205, w19204, w19203, w19202, w19201, w19200, w19199, w19198, w19197, w19196, w19195, w19194) -> (w19223:dbl[])
              }
              frame 1 {
                n7503 = Unbundle By Name(w19277) -> ("充电结束电压(90%)"=w19261:sgl, "充电结束电压(91%)"=w19260:sgl, "充电结束电压(92%)"=w19259:sgl, "充电结束电压(93%)"=w19258:sgl, "充电结束电压(94%)"=w19257:sgl, "充电结束电压(95%)"=w19256:sgl, "充电结束电压(96%)"=w19255:sgl, "充电结束电压(97%)"=w19254:sgl, "充电结束电压(98%)"=w19253:sgl, "充电结束电压(99%)"=w19252:sgl, "充电结束电压(100%)"=w19251:sgl)
                n7504 = call "输入分辨率计算-EV05.vi"("1字节?"=FALSE, "数值 2"=w19258, "数值"=w19259, "分辨率"=0.001) -> ("低字节 2"=w19242:dbl, "高字节 2"=w19243:dbl, "低字节"=w19244:dbl, "高字节1"=w19245:dbl)  [unwired: 1 in, 3 out]
                n7505 = call "输入分辨率计算-EV05.vi"("1字节?"=FALSE, "数值 2"=w19256, "数值"=w19257, "分辨率"=0.001) -> ("低字节 2"=w19238:dbl, "高字节 2"=w19239:dbl, "低字节"=w19240:dbl, "高字节1"=w19241:dbl)  [unwired: 1 in, 3 out]
                n7506 = call "输入分辨率计算-EV05.vi"("1字节?"=FALSE, "数值"=w19251, "分辨率"=0.001) -> ("低字节"=w19228:dbl, "高字节1"=w19229:dbl)  [unwired: 2 in, 5 out]
                n7507 = call "输入分辨率计算-EV05.vi"("1字节?"=FALSE, "数值 2"=w19252, "数值"=w19253, "分辨率"=0.001) -> ("低字节 2"=w19230:dbl, "高字节 2"=w19231:dbl, "低字节"=w19232:dbl, "高字节1"=w19233:dbl)  [unwired: 1 in, 3 out]
                n7508 = call "输入分辨率计算-EV05.vi"("1字节?"=FALSE, "数值 2"=w19260, "数值"=w19261, "分辨率"=0.001) -> ("低字节 2"=w19246:dbl, "高字节 2"=w19247:dbl, "低字节"=w19248:dbl, "高字节1"=w19250:dbl)  [unwired: 1 in, 3 out]
                n7509 = call "输入分辨率计算-EV05.vi"("1字节?"=FALSE, "数值 2"=w19254, "数值"=w19255, "分辨率"=0.001) -> ("低字节 2"=w19234:dbl, "高字节 2"=w19235:dbl, "低字节"=w19236:dbl, "高字节1"=w19237:dbl)  [unwired: 1 in, 3 out]
                n7510 = Build Array(w19250, w19248, w19247, w19246, w19245, w19244, w19243, w19242, w19241, w19240, w19239, w19238, w19237, w19236, w19235, w19234, w19233, w19232, w19231, w19230, w19229, w19228) -> (w19249:dbl[])
              }
            }
          }
        }
        frame "充电结束电压" {
          w19281 = 1
          n7511 = Unbundle By Name(w19284) -> ("均衡参数"=w19279:refnum<vi>)
          n7512 = property class="Clust (严格)"(reference=w19279) -> ("Value"=w19278:T10)  [unwired: 1 in, 2 out]
          n7513 = for {
            N: w19281 -> [_]
            tunnel: [w19292] -> w19286 mode=indexing
            tunnel: [w19291] -> w19285 mode=indexing
            tunnel: w19278 -> [w19290]
            tunnel: [w19289] -> w19283 mode=indexing
            tunnel: [w19287] -> w19280 mode=indexing
            i -> [w19288]
            n7514 = case shown="0, 默认" w19288 {
              tunnel: [22 ("单个参数补充") 24 ("命令序号")] -> w19292
              tunnel: [u32 2 ("命令序号") u32 1 ("命令序号")] -> w19291
              tunnel: w19290 -> [w19342 w19373]
              tunnel: [w19314 w19372] -> w19289
              tunnel: ["充电结束电压" "均衡阀值"] -> w19287
              frame 0, Default {
                n7515 = Unbundle By Name(w19342) -> ("充电结束电压(90%)"=w19326:sgl, "充电结束电压(91%)"=w19325:sgl, "充电结束电压(92%)"=w19324:sgl, "充电结束电压(93%)"=w19323:sgl, "充电结束电压(94%)"=w19322:sgl, "充电结束电压(95%)"=w19321:sgl, "充电结束电压(96%)"=w19320:sgl, "充电结束电压(97%)"=w19319:sgl, "充电结束电压(98%)"=w19318:sgl, "充电结束电压(99%)"=w19317:sgl, "充电结束电压(100%)"=w19316:sgl)
                n7516 = call "输入分辨率计算-EV05.vi"("1字节?"=FALSE, "数值 2"=w19323, "数值"=w19324, "分辨率"=0.001) -> ("低字节 2"=w19307:dbl, "高字节 2"=w19308:dbl, "低字节"=w19309:dbl, "高字节1"=w19310:dbl)  [unwired: 1 in, 3 out]
                n7517 = call "输入分辨率计算-EV05.vi"("1字节?"=FALSE, "数值 2"=w19321, "数值"=w19322, "分辨率"=0.001) -> ("低字节 2"=w19303:dbl, "高字节 2"=w19304:dbl, "低字节"=w19305:dbl, "高字节1"=w19306:dbl)  [unwired: 1 in, 3 out]
                n7518 = call "输入分辨率计算-EV05.vi"("1字节?"=FALSE, "数值"=w19316, "分辨率"=0.001) -> ("低字节"=w19293:dbl, "高字节1"=w19294:dbl)  [unwired: 2 in, 5 out]
                n7519 = call "输入分辨率计算-EV05.vi"("1字节?"=FALSE, "数值 2"=w19317, "数值"=w19318, "分辨率"=0.001) -> ("低字节 2"=w19295:dbl, "高字节 2"=w19296:dbl, "低字节"=w19297:dbl, "高字节1"=w19298:dbl)  [unwired: 1 in, 3 out]
                n7520 = call "输入分辨率计算-EV05.vi"("1字节?"=FALSE, "数值 2"=w19325, "数值"=w19326, "分辨率"=0.001) -> ("低字节 2"=w19311:dbl, "高字节 2"=w19312:dbl, "低字节"=w19313:dbl, "高字节1"=w19315:dbl)  [unwired: 1 in, 3 out]
                n7521 = call "输入分辨率计算-EV05.vi"("1字节?"=FALSE, "数值 2"=w19319, "数值"=w19320, "分辨率"=0.001) -> ("低字节 2"=w19299:dbl, "高字节 2"=w19300:dbl, "低字节"=w19301:dbl, "高字节1"=w19302:dbl)  [unwired: 1 in, 3 out]
                n7522 = Build Array(w19315, w19313, w19312, w19311, w19310, w19309, w19308, w19307, w19306, w19305, w19304, w19303, w19302, w19301, w19300, w19299, w19298, w19297, w19296, w19295, w19294, w19293) -> (w19314:dbl[])
              }
              frame 1 {
                n7523 = Unbundle By Name(w19373) -> ("均衡计算-电压高阀值1级"=w19363:sgl, "均衡计算-电压高阀值2级"=w19362:sgl, "均衡计算-电压低阀值1级"=w19361:sgl, "均衡计算-电压低阀值2级"=w19360:sgl, "均衡计算-最低电压阀值"=w19359:sgl, "均衡停止-最低电压阀值"=w19358:sgl, "均衡计算-电压极差阀值"=w19357:sgl)
                n7524 = call "输入分辨率计算-EV05.vi"("1字节?"=FALSE, "数值"=w19357, "分辨率"=0.001) -> ("低字节"=w19343:dbl, "高字节1"=w19344:dbl)  [unwired: 2 in, 5 out]
                n7525 = call "输入分辨率计算-EV05.vi"("1字节?"=FALSE, "数值 2"=w19358, "数值"=w19359, "分辨率"=0.001) -> ("低字节 2"=w19345:dbl, "高字节 2"=w19346:dbl, "低字节"=w19347:dbl, "高字节1"=w19348:dbl)  [unwired: 1 in, 3 out]
                n7526 = call "输入分辨率计算-EV05.vi"("1字节?"=FALSE, "数值 2"=w19362, "数值"=w19363, "分辨率"=0.001) -> ("低字节 2"=w19353:dbl, "高字节 2"=w19354:dbl, "低字节"=w19355:dbl, "高字节1"=w19356:dbl)  [unwired: 1 in, 3 out]
                n7527 = call "输入分辨率计算-EV05.vi"("1字节?"=FALSE, "数值 2"=w19360, "数值"=w19361, "分辨率"=0.001) -> ("低字节 2"=w19349:dbl, "高字节 2"=w19350:dbl, "低字节"=w19351:dbl, "高字节1"=w19352:dbl)  [unwired: 1 in, 3 out]
                n7528 = Build Array(w19356, w19355, w19354, w19353, w19352, w19351, w19350, w19349, w19348, w19347, w19346, w19345, w19344, w19343) -> (w19372:dbl[])
              }
            }
          }
        }
        frame "电池包信息1" {
          n7529 = case shown="真" w19380 {
            tunnel: [_ w19393] -> w19384
            tunnel: [_ w19392] -> w19383
            tunnel: w19382 -> [_ w19388]
            tunnel: [_ w19391] -> w19381
            tunnel: [_ u32 35 ("命令序号")] -> w19379
            tunnel: [_ w19386] -> w19378
            tunnel: [_ w19385] -> w19377
            frame False {
            }
            frame True {
              w19386 = 1
              n7530 = Unbundle By Name(w19388) -> ("电池组信息(从板)"=w19389:refnum<vi>)
              n7531 = property class="Clust (严格)"(reference=w19389) -> ("Value"=w19387:T9)  [unwired: 1 in, 2 out]
              n7532 = for {
                N: w19386 -> [_]
                tunnel: [w19399] -> w19393 mode=indexing
                tunnel: [w19398] -> w19392 mode=indexing
                tunnel: w19387 -> [w19397]
                tunnel: [w19396] -> w19391 mode=indexing
                tunnel: [w19394] -> w19385 mode=indexing
                i -> [w19395]
                n7533 = case shown="0, 默认" w19395 {
                  tunnel: [30 ("单个参数补充") 4 ("单个参数补充") 8 ("单个参数补充") 6 ("单个参数补充") 4 ("单个参数补充") 8 ("单个参数补充") 14 ("单个参数补充")] -> w19399
                  tunnel: [u32 1 ("命令序号") u32 2 ("命令序号") u32 3 ("命令序号") u32 4 ("命令序号") u32 5 ("命令序号") u32 6 ("命令序号") u32 7 ("命令序号")] -> w19398
                  tunnel: w19397 -> [w19403 w19478 w19486 w19516 w19527 w19535 w19556]
                  tunnel: [w19400 w19471 w19503 w19518 w19528 w19533 w19558] -> w19396
                  tunnel: ["电池包信息1" "电池包序号" "充放电安时" "充电次数时间" "SOC" "车牌号" "充电参数"] -> w19394
                  frame 0, Default {
                    w19413 = ":" ("正则表达式")
                    w19421 = 0.0 ("元素")
                    w19440 = 256.0 ("y")
                    w19445 = 256.0 ("y")
                    w19458 = 2 ("偏移量(0)")
                    w19455 = "-" ("正则表达式")
                    # "电池组信息"
                    n7534 = Unbundle By Name(w19403) -> ("串联数"=w19462:dbl, "并联数"=w19461:dbl, "电池厂家"=w19401:dbl, "电池类型"=w19402:dbl, "生产日期"=w19460:string)
                    n7535 = Unbundle By Name(w19403) -> ("额定能量"=w19426:dbl, "额定容量"=w19428:dbl, "实际容量"=w19427:dbl, "额定总压"=w19451:dbl)
                    n7536 = Match Pattern(string=w19460, regular expression=w19455) -> (before substring=w19459:string, after substring=w19456:string)  [unwired: 3 out]
                    n7537 = Match Pattern(string=w19456, regular expression=w19455) -> (before substring=w19454:string, after substring=w19419:string)  [unwired: 3 out]
                    n7538 = Match Pattern(string=w19419, regular expression=" " ("正则表达式")) -> (before substring=w19417:string, after substring=w19416:string)  [unwired: 3 out]
                    n7539 = call "输入分辨率计算-EV05.vi"("1字节?"=FALSE, "数值"=w19426, "分辨率"=0.1) -> ("低字节"=w19425:dbl, "高字节1"=w19424:dbl)  [unwired: 2 in, 5 out]
                    n7540 = String Subset(string=w19459, offset (0)=w19458, length (rest)=w19458) -> (substring=w19457:string)
                    n7541 = call "输入分辨率计算-EV05.vi"("1字节?"=TRUE, "数值 2"=w19427, "数值"=w19428, "分辨率"=0.001) -> ("高字节 2"=w19429:dbl, "高字节1"=w19430:dbl)  [unwired: 1 in, 5 out]
                    n7542 = Match Pattern(string=w19416, regular expression=w19413) -> (before substring=w19415:string, after substring=w19414:string)  [unwired: 3 out]
                    n7543 = Fract/Exp String To Number(string=w19457) -> (number=w19409:dbl)  [unwired: 1 in, 3 out]
                    n7544 = Fract/Exp String To Number(string=w19454) -> (number=w19408:dbl)  [unwired: 4 out]
                    n7545 = Fract/Exp String To Number(string=w19417) -> (number=w19407:dbl)  [unwired: 4 out]
                    n7546 = Match Pattern(string=w19414, regular expression=w19413) -> (before substring=w19412:string, after substring=w19411:string)  [unwired: 3 out]
                    n7547 = call "输入分辨率计算-EV05.vi"("1字节?"=FALSE, "数值"=w19451, "分辨率"=0.1) -> ("低字节"=w19422:dbl, "高字节1"=w19423:dbl)  [unwired: 2 in, 5 out]
                    n7548 = Quotient & Remainder(x=w19430, y=w19445) -> (x-y*floor(x/y)=w19444:dbl, floor(x/y)=w19448:dbl)
                    n7549 = Fract/Exp String To Number(string=w19415) -> (number=w19406:dbl)  [unwired: 4 out]
                    n7550 = Quotient & Remainder(x=w19429, y=w19440) -> (x-y*floor(x/y)=w19436:dbl, floor(x/y)=w19437:dbl)
                    n7551 = Quotient & Remainder(x=w19448, y=w19445) -> (x-y*floor(x/y)=w19443:dbl, floor(x/y)=w19447:dbl)
                    n7552 = Fract/Exp String To Number(string=w19412) -> (number=w19405:dbl)  [unwired: 4 out]
                    n7553 = Quotient & Remainder(x=w19437, y=w19440) -> (x-y*floor(x/y)=w19435:dbl, floor(x/y)=w19438:dbl)
                    n7554 = call <vilib>:"Trim Whitespace.vi"("string"=w19411) -> ("trimmed string"=w19410:string)  [unwired: 1 in]
                    n7555 = Quotient & Remainder(x=w19447, y=w19445) -> (x-y*floor(x/y)=w19442:dbl, floor(x/y)=w19446:dbl)
                    n7556 = Quotient & Remainder(x=w19438, y=w19440) -> (x-y*floor(x/y)=w19434:dbl, floor(x/y)=w19439:dbl)
                    n7557 = Quotient & Remainder(x=w19462, y=256.0) -> (x-y*floor(x/y)=w19464:dbl, floor(x/y)=w19465:dbl)
                    n7558 = Fract/Exp String To Number(string=w19410) -> (number=w19404:dbl)  [unwired: 4 out]
                    n7559 = Quotient & Remainder(x=w19446, y=w19445) -> (x-y*floor(x/y)=w19441:dbl)  [unwired: 1 out]
                    n7560 = Quotient & Remainder(x=w19439, y=w19440) -> (x-y*floor(x/y)=w19433:dbl)  [unwired: 1 out]
                    n7561 = Build Array(w19424, w19425, w19441, w19442, w19443, w19444, w19433, w19434, w19435, w19436, w19423, w19422, w19421, w19421, w19421, w19409, w19408, w19407, w19406, w19405, w19404) -> (w19420:dbl[])
                    n7562 = Build Array(w19465, w19464, w19461, w19401, w19402) -> (w19463:dbl[])
                    n7563 = Insert Into Array(array=w19463, new element=w19420) -> (w19400:dbl[])  [unwired: 1 in]
                  }
                  frame 1 {
                    n7564 = Unbundle By Name(w19478) -> ("电池包序号"=w19475:dbl)
                    n7565 = Quotient & Remainder(x=w19475, y=256.0) -> (x-y*floor(x/y)=w19472:dbl, floor(x/y)=w19473:dbl)
                    n7566 = Build Array(w19473, w19472) -> (w19471:dbl[])
                  }
                  frame 2 {
                    w19494 = 256.0 ("y")
                    w19499 = 256.0 ("y")
                    # "充放电安时/安时数"
                    n7567 = Unbundle By Name(w19486) -> ("充电总安时"=w19483:dbl, "放电总这时"=w19482:dbl)
                    n7568 = call "输入分辨率计算-EV05.vi"("1字节?"=TRUE, "数值 2"=w19482, "数值"=w19483, "分辨率"=0.001) -> ("高字节 2"=w19480:dbl, "高字节1"=w19481:dbl)  [unwired: 1 in, 5 out]
